vi "Read Measurement (Multiple).vi"(8 "error in (no error)":errorcluster, 9 "Timeout (10000 ms)":i32=10000, 10 "Number of Measurements (1)":i32=1, 11 "VISA resource name":refnum<visa-resource-name>) -> (0 "error out":errorcluster, 2 "Measurements":dbl[](array[numeric]), 3 "VISA resource name out":refnum<visa-resource-name>)   [LabVIEW 2019, in "Pendulum CNT90.lvlib"]
doc: "The read function performs new measurements and reads out a measuring array of results."
uses:
  Pendulum CNT90.lvlib
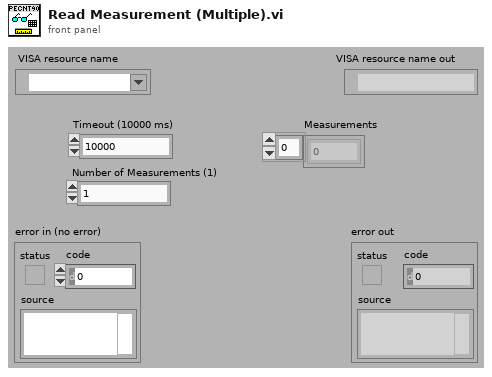
[diagram p1: front panel]
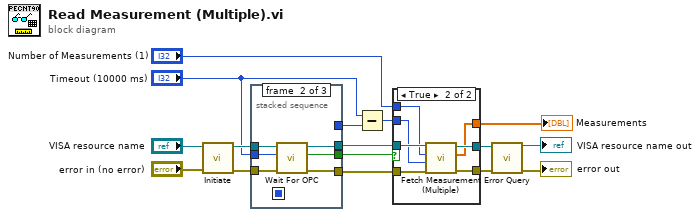
[diagram p0: block diagram]
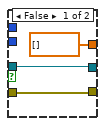
[diagram p2: hidden frame]
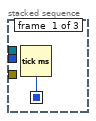
[diagram p3: hidden frame]
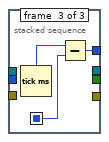
[diagram p4: hidden frame]
diagram:
  n1 = call "Initiate.vi"("error in (no error)"="error in (no error)", "VISA resource name"="VISA resource name") -> ("error out"=w8:errorcluster, "VISA resource name out"=w9:refnum<visa-resource-name>)  [unwired: 8 in]
  n2 = stacked-sequence {
    seq-local: [w17 _ _] -> [_ _ w25]
    tunnel: w9 -> [_ w20 _]
    tunnel: w8 -> [_ w21 _]
    tunnel: [_ w22 _] -> w6
    tunnel: [_ w23 _] -> w7
    tunnel: [_ _ w24] -> w5
    tunnel: [_ w19 _] -> w3
    tunnel: "Timeout (10000 ms)" -> [_ w18 _]
    frame #0 {
      n3 = Tick Count (ms)() -> (millisecond timer value=w17:u32)
    }
    frame #1 {
      n4 = call "Wait For OPC.vi"("error in (no error)"=w21, "Timeout (10000 ms)"=w18, "VISA resource name"=w20) -> ("error out"=w22:errorcluster, "Complete"=w19:bool, "VISA resource name out"=w23:refnum<visa-resource-name>)  [unwired: 6 in]
    }
    frame #2 {
      n5 = Tick Count (ms)() -> (millisecond timer value=w26:u32)
      n6 = Subtract(x=w26, y=w25) -> (x-y=w24:u32)
    }
  }
  n7 = Subtract(x="Timeout (10000 ms)", y=w5) -> (x-y=w2:u32)
  n8 = case shown="True" w3 {
    tunnel: [w29 w36] -> w12
    tunnel: [w28 w35] -> w11
    tunnel: [dbl[] [] ("Results") w34] -> w10
    tunnel: w7 -> [w29 w33]
    tunnel: w6 -> [w28 w32]
    tunnel: w2 -> [_ w31]
    tunnel: "Number of Measurements (1)" -> [_ w30]
    frame False {
    }
    frame True {
      n9 = call "Fetch Measurement (Multiple).vi"("error in (no error)"=w32, "Timeout (10000 ms)"=w31, "Number of Measurements (1)"=w30, "VISA resource name"=w33) -> ("error out"=w35:errorcluster, "Measurements"=w34:dbl[], "VISA resource name out"=w36:refnum<visa-resource-name>)  [unwired: 5 in]
    }
  }
  "Measurements" <- w10
  n10 = call "Error Query.vi"("error in (no error)"=w11, "VISA resource name"=w12) -> ("error out"=→"error out":errorcluster, "VISA resource name out"=→"VISA resource name out":refnum<visa-resource-name>)  [unwired: 6 in, 2 out]
